vi "Start Log.vi"(8 "error in (no error)":errorcluster, 11 "Historian Logger in":refnum<class "Historian Logger.lvclass">) -> (0 "error out":errorcluster, 3 "Historian Logger out":refnum<class "Historian Logger.lvclass">)   [LabVIEW 2020, in "VolatusHistorian.lvlib" / "Historian Logger.lvclass"]
uses:
  Historian Logger.lvclass
  Historian Logger.lvclass/Historian Logger.ctl
  lv-cdm/CDM-Config/CDM-Config.lvlib
  lv-cdm/CDM-Config/Format.ctl
  lv-cdm/CDM-Config/Precision.ctl
  lv-cdm/CDM-Config/Timezone.ctl
  lv-cdm/CDM-Config/ISO8601 Config.ctl
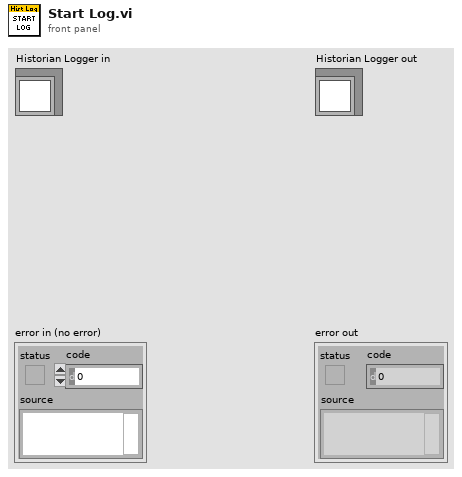
[diagram p1: front panel]
types:
  T1 = typedef "CDM-Config.lvlib/ISO8601 Config.ctl" = cluster{"Format":T2, "Precision":T3, "Timezone":T4}
  T2 = typedef "CDM-Config.lvlib/Format.ctl" = enum16{"Extended", "Basic"}
  T3 = typedef "CDM-Config.lvlib/Precision.ctl" = enum16{"Millisecond", "Second", "Minute", "Hour", "Day"}
  T4 = typedef "CDM-Config.lvlib/Timezone.ctl" = enum16{"UTC", "Local"}
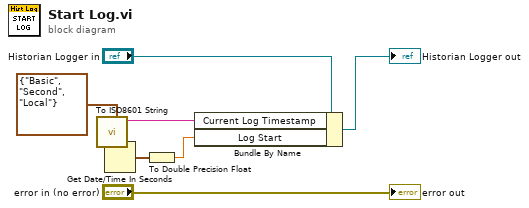
[diagram p0: block diagram]
diagram:
  n1 = call "To ISO8601 String.vi"("Format Config"=T1 {"Format"=enum."Basic", "Precision"=enum."Second", "Timezone"=enum."Local"}) -> ("ISO 8601"=w3:string)  [unwired: 10 in]
  n2 = Get Date/Time In Seconds() -> (seconds since 1Jan1904=w2:timestamp)
  n3 = To Double Precision Float(number=w2) -> (double precision float=w1:dbl)
  n4 = Bundle By Name(cluster="Historian Logger in", "Current Log Timestamp"=w3, "Log Start"=w1) -> (→"Historian Logger out":refnum<class "Historian Logger.lvclass">)
  "error out" <- "error in (no error)"
